vi "ClassPanel.vi"(8 "error in (no error)":errorcluster caption="entrée d'erreur (pas d'erreur)", 11 "RedTide650.lvclass":refnum<class "RedTide650.lvclass">) -> (0 "error out":errorcluster caption="sortie d'erreur", 3 "RedTide650.lvclass Out":refnum<class "RedTide650.lvclass">)   [LabVIEW 2019, in "RedTide650.lvclass"]
uses:
  RedTide650.lvclass
  C:/Programmes Labview/LabScanV1A/DevicesClass/BaseDevice/BaseDevice.lvclass
  BaseDevice/ClassQueueMess.ctl
  RedTide650.lvclass/RedTide650.ctl
  BaseDevice/Accessor/GetClassEvent.vi
panel:
  in  "Save Data":bool caption="Save\nData"
  in  "Data File Path":path
  in  "MainProgQ":refnum<queue>
  in  "MainProgQEvent":refnum<user-event>
  in  "Acq":bool
  in  "Stop":bool
  out "Filename":string
  in  "Acquire":bool caption="MiseAJour"
  in  "FileIndex":u32=60 min=1 step=1
  out "Init Program":bool
  # "Red Tide USB650"
  # "this MUST labeled with class name"
  # "this MUST be present and labeled \"Stop\" and \"Acq\""
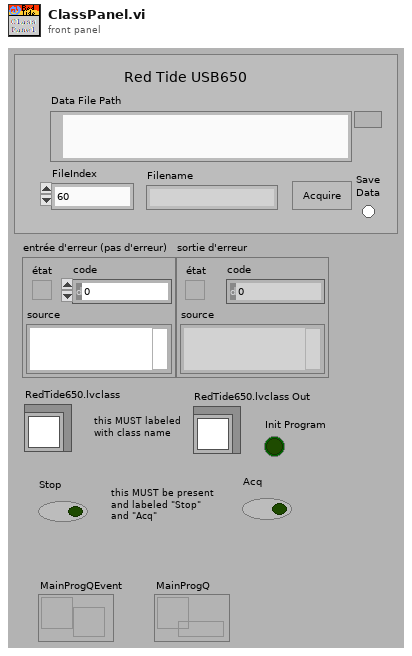
[diagram p1: front panel]
types:
  T1 = typedef "ClassQueueMess.ctl" = u16
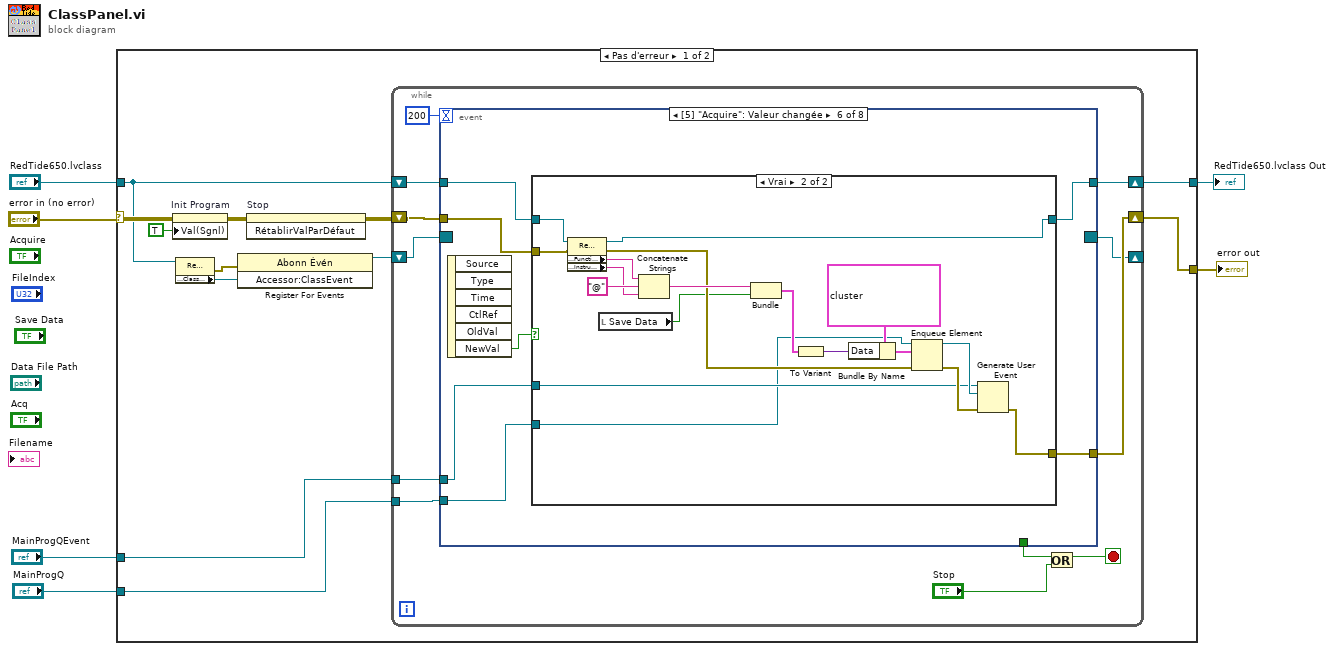
[diagram p0: block diagram]
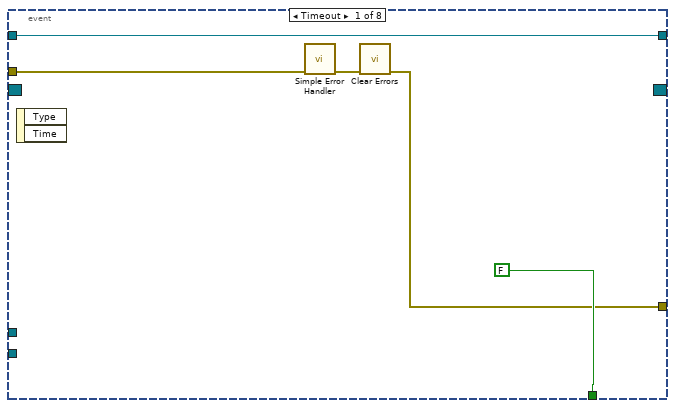
[diagram p2: hidden frame]
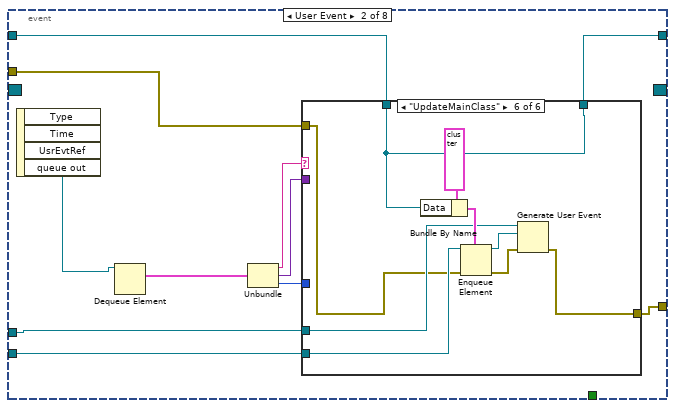
[diagram p3: hidden frame]
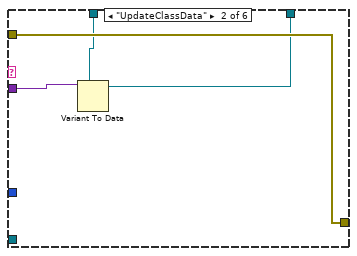
[diagram p5: hidden frame]
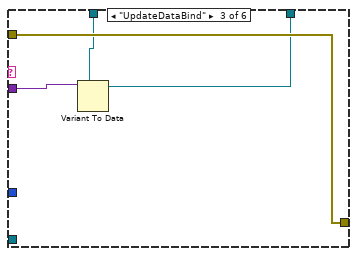
[diagram p6: hidden frame]
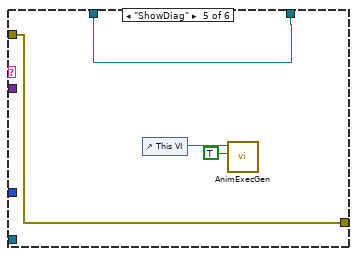
[diagram p8: hidden frame]
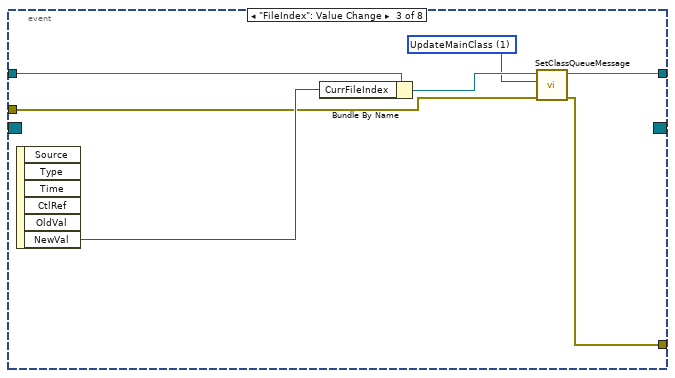
[diagram p9: hidden frame]
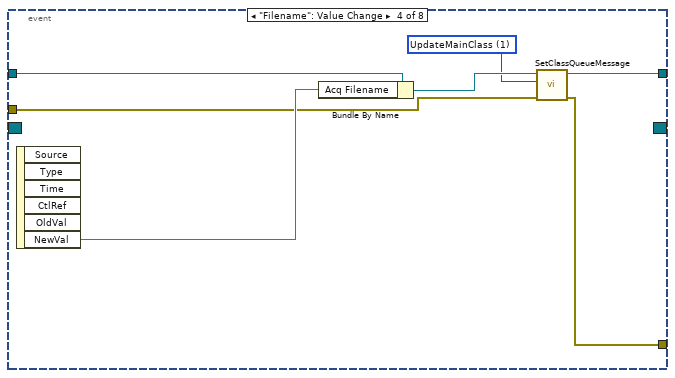
[diagram p10: hidden frame]
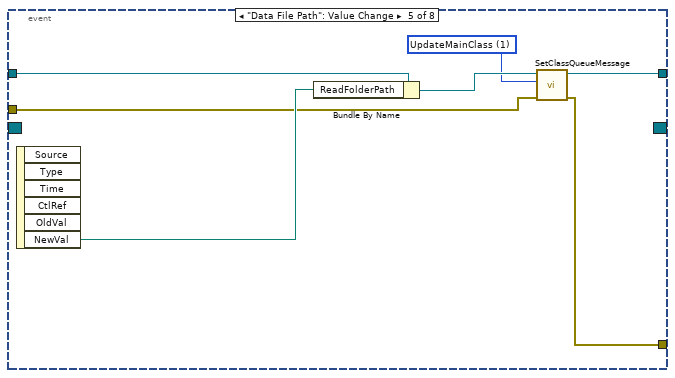
[diagram p11: hidden frame]
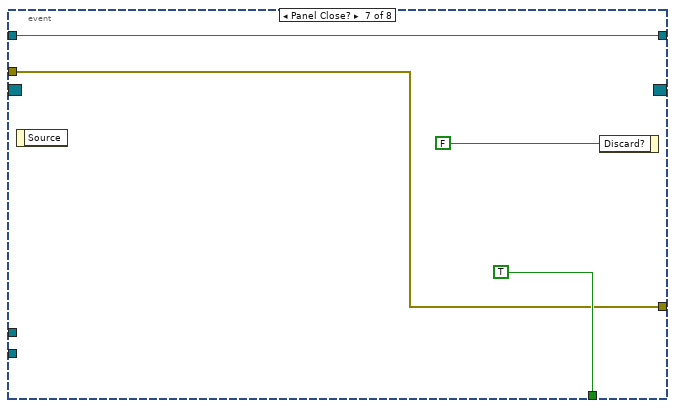
[diagram p13: hidden frame]
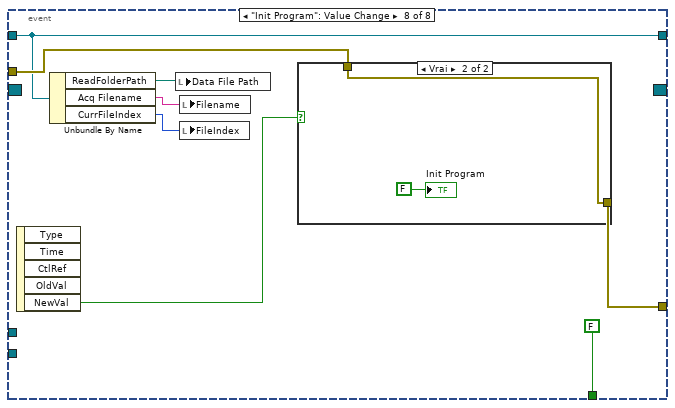
[diagram p14: hidden frame]
diagram:
  n1 = case shown="Pas d'erreur" "error in (no error)" {
    selector: "error in (no error)" -> [w15 w136]
    tunnel: [w18 w136] -> w5
    tunnel: "RedTide650.lvclass" -> [w10 w135]
    tunnel: [w16 w135] -> w3
    tunnel: "MainProgQEvent" -> [w8 _]
    tunnel: "MainProgQ" -> [w7 _]
    frame No Error {
      n2 = property on="Init Program" class="Bool (strict)"(error in=w15, "Val(Sgnl)"=TRUE ("Valeur (Signalisation)")) -> (error out=w14:errorcluster)  [unwired: 1 in, 1 out]
      n3 = property class="RedTide650.lvclass"(reference=w10) -> (error out=w12:errorcluster, "Accessor:ClassEvent"=w11:refnum<user-event>)  [unwired: 1 in, 1 out]
      n4 = register-events(error in=w12, w11) -> (reference out=w9:refnum<event-registration>)  [unwired: 1 in, 1 out]
      n5 = invoke on="Stop" class="Bool (strict)" method="RétablirValParDéfaut"(error in=w14) -> (error out=w13:errorcluster)  [unwired: 2 in, 2 out]
      n6 = while {
        shift-right: [w28] -> w18
        shift-left: w13 -> [w29]
        shift-right: [w25] -> w16
        shift-left: w10 -> [w27]
        shift-right: [w21] -> _
        shift-left: w9 -> [w22]
        tunnel: w8 -> [w20]
        tunnel: w7 -> [w19]
        stop <- w24 stop-if-true
        n7 = event shown="[5] \"Acquire\": Valeur changée" {
          selector: w22 -> [_ _ _ _ _ _ _ _]
          dyn-events: [_ _ _ _ _ _ _ _] -> w21
          timeout: 200 -> [_ _ _ _ _ _ _ _]
          tunnel: w29 -> [w33 w45 w74 w81 w88 w96 w121 w130]
          tunnel: [w31 w39 w73 w80 w87 w94 w121 w129] -> w28
          tunnel: w27 -> [w34 w46 w78 w85 w92 w93 w120 w127]
          tunnel: [FALSE _ _ _ _ _ TRUE FALSE] -> w26
          tunnel: [w34 w38 w75 w82 w89 w98 w120 w127] -> w25
          tunnel: w20 -> [_ w37 _ _ _ w97 _ _]
          tunnel: w19 -> [_ w36 _ _ _ w95 _ _]
          event Timeout {
            n8 = event-data() -> ()  [unwired: 1 in, 2 out]
            n9 = call <vilib>:"Simple Error Handler.vi"("error in (no error)"=w33) -> ("error out"=w32:errorcluster)  [unwired: 4 in, 4 out]
            n10 = call <vilib>:"Clear Errors.vi"("error in (no error)"=w32) -> ("error out"=w31:errorcluster)  [unwired: 5 in, 1 out]
          }
          event User Event {
            n11 = event-data() -> ("queue out"=w43:refnum<queue>)  [unwired: 1 in, 3 out]
            n12 = Dequeue Element(queue=w43) -> (element=w44:cluster{"Message":string, "Data":variant, i32})  [unwired: 2 in, 3 out]
            n13 = Unbundle(w44) -> ("Message"=w42:string, "Data"=w41:variant, w40:i32)
            n14 = case shown="\"UpdateMainClass\"" w42 {
              tunnel: w45 -> [w48 w52 w56 w57 w61 w64]
              tunnel: w41 -> [_ w51 w55 _ _ _]
              tunnel: w46 -> [w47 w50 w54 w58 w62 w67]
              tunnel: [w47 w49 w53 w58 w62 w67] -> w38
              tunnel: [w48 w52 w56 w57 w61 w63] -> w39
              tunnel: w40 -> [_ _ _ _ _ _]
              tunnel: w37 -> [_ _ _ _ _ w66]
              tunnel: w36 -> [_ _ _ _ _ w65]
              frame Default {
              }
              frame "UpdateClassData" {
                n15 = Variant To Data(type=w50, Variant=w51) -> (data=w49:refnum<class "RedTide650.lvclass">)  [unwired: 1 in, 1 out]
              }
              frame "UpdateDataBind" {
                n16 = Variant To Data(type=w54, Variant=w55) -> (data=w53:refnum<class "RedTide650.lvclass">)  [unwired: 1 in, 1 out]
              }
              frame "MeasDone" {
              }
              frame "ShowDiag" {
                n17 = control-ref of="This VI"() -> (w60:refnum<vi>)
                n18 = call <userlib>:"AnimExecGen.vi"("Animer l'exécution ?"=TRUE, "ViRef"=w60) -> ()  [unwired: 9 in, 1 out]
              }
              frame "UpdateMainClass" {
                n19 = Bundle By Name(cluster=cluster{"Message":string, "Data":variant, i32} {"Message"="", "Data"=variant, 0} ("élément"), "Data"=w67) -> (w68:cluster{"Message":string, "Data":variant, i32})
                n20 = Enqueue Element(queue=w65, element=w68, error in (no error)=w64) -> (queue out=w71:refnum<queue>, error out=w70:errorcluster)  [unwired: 1 in, 1 out]
                n21 = Generate User Event(user event=w66, event data cluster=w71, error in=w70) -> (error out=w63:errorcluster)  [unwired: 1 in, 1 out]
              }
            }
          }
          event "FileIndex": Value Change {
            w72 = T1 1 items=["UpdateClassData", "UpdateMainClass", "UpdateDataBind", "ReInitDevice", "Custom", "ClosePan"] ("Menu déroulant")
            n22 = event-data() -> ("NewVal"=w77:u32)  [unwired: 1 in, 5 out]
            n23 = Bundle By Name(cluster=w78, "CurrFileIndex"=w77) -> (w76:refnum<class "RedTide650.lvclass">)
            n24 = call-dynamic "SetClassQueueMessage.vi"("ErrorIn(No Error)"=w74, "Menu déroulant"=w72, "DefaultDev.lvclass"=w76) -> ("sortie d'erreur"=w73:errorcluster, "DefaultDev.lvclass Out"=w75:refnum<class "RedTide650.lvclass">)  [unwired: 7 in]
          }
          event "Filename": Value Change {
            w79 = T1 1 items=["UpdateClassData", "UpdateMainClass", "UpdateDataBind", "ReInitDevice", "Custom", "ClosePan"] ("Menu déroulant")
            n25 = event-data() -> ("NewVal"=w84:string)  [unwired: 1 in, 5 out]
            n26 = Bundle By Name(cluster=w85, "Acq Filename"=w84) -> (w83:refnum<class "RedTide650.lvclass">)
            n27 = call-dynamic "SetClassQueueMessage.vi"("ErrorIn(No Error)"=w81, "Menu déroulant"=w79, "DefaultDev.lvclass"=w83) -> ("sortie d'erreur"=w80:errorcluster, "DefaultDev.lvclass Out"=w82:refnum<class "RedTide650.lvclass">)  [unwired: 7 in]
          }
          event "Data File Path": Value Change {
            w86 = T1 1 items=["UpdateClassData", "UpdateMainClass", "UpdateDataBind", "ReInitDevice", "Custom", "ClosePan"] ("Menu déroulant")
            n28 = event-data() -> ("NewVal"=w91:path)  [unwired: 1 in, 5 out]
            n29 = Bundle By Name(cluster=w92, "ReadFolderPath"=w91) -> (w90:refnum<class "RedTide650.lvclass">)
            n30 = call-dynamic "SetClassQueueMessage.vi"("ErrorIn(No Error)"=w88, "Menu déroulant"=w86, "DefaultDev.lvclass"=w90) -> ("sortie d'erreur"=w87:errorcluster, "DefaultDev.lvclass Out"=w89:refnum<class "RedTide650.lvclass">)  [unwired: 7 in]
          }
          event "Acquire": Value Change {
            n31 = event-data() -> ("NewVal"=w99:bool)  [unwired: 1 in, 5 out]
            n32 = case shown="Vrai" w99 {
              tunnel: [w101 w106] -> w98
              tunnel: w93 -> [w101 w107]
              tunnel: w97 -> [_ w114]
              tunnel: w96 -> [w100 w109]
              tunnel: w95 -> [_ w104]
              tunnel: [w100 w103] -> w94
              frame False {
              }
              frame True {
                n33 = property class="RedTide650.lvclass"(reference=w107, error in=w109) -> (reference out=w106:refnum<class "RedTide650.lvclass">, error out=w108:errorcluster, "Accessor:Function"=w113:string, "Accessor:InstrumentName"=w111:string)
                n34 = local read "Save Data"() -> (w102:bool)
                n35 = Concatenate Strings(w113, "@" ("chaîne"), w111) -> (w110:string)
                n36 = Bundle(w110, "Save Data"=w102) -> (w105:cluster{string, "Save Data":bool})  [unwired: 1 in]
                n37 = To Variant(anything=w105) -> (Variant=w117:variant)
                n38 = Bundle By Name(cluster=cluster{"Message":string, "Data":variant, i32} {"Message"="ArrayDevAcqSetup", "Data"=variant, 0} ("élément"), "Data"=w117) -> (w116:cluster{"Message":string, "Data":variant, i32})
                n39 = Enqueue Element(queue=w104, element=w116, error in (no error)=w108) -> (queue out=w119:refnum<queue>, error out=w115:errorcluster)  [unwired: 1 in, 1 out]
                n40 = Generate User Event(user event=w114, event data cluster=w119, error in=w115) -> (error out=w103:errorcluster)  [unwired: 1 in, 1 out]
              }
            }
          }
          event Panel Close? {
            n41 = event-data() -> ()  [unwired: 1 in, 1 out]
            n42 = event-data("Discard?"=FALSE ("Rejeter ?")) -> ()  [unwired: 1 in, 1 out]
          }
          event "Init Program": Value Change {
            n43 = event-data() -> ("NewVal"=w131:bool)  [unwired: 1 in, 4 out]
            n44 = Unbundle By Name(w127) -> ("ReadFolderPath"=w124:path, "Acq Filename"=w126:string, "CurrFileIndex"=w125:u32)
            n45 = local write "Data File Path"(w124) -> ()
            n46 = local write "Filename"(w126) -> ()
            n47 = local write "FileIndex"(w125) -> ()
            n48 = case shown="Vrai" w131 {
              tunnel: w130 -> [w132 w133]
              tunnel: [w132 w133] -> w129
              frame False {
              }
              frame True {
                "Init Program" <- FALSE
              }
            }
          }
        }
        n49 = Or(x=w26, y="Stop") -> (x .or. y?=w24:bool)
      }
    }
    frame Error {
    }
  }
  "error out" <- w5
  "RedTide650.lvclass Out" <- w3
